vi "adapt_image_report.vi"() -> (3 "adapted image":T1)   [LabVIEW 2011]
doc: "Crops an image (original or captured) to cubic format (x-resolution = y-resolution) and applies a circular mask. Cropping and masking can be corrected using the crop-correction and mask-correction inputs.\n\nIf the input image is original (captured image set to FALSE) the image size will be adapted to match the size of the captured image and the image is flipped along the horizontal axis to account for the mirror image."
uses:
  <vilib>/vision/Image Controls.llb/IMAQ Image.ctl
  global_vars.vi
  <vilib>/vision/NI_Vision_Development_Module.lvlib
panel:
  out "cropped":T1(plugin-control)
  out "resized":T1(plugin-control)
  out "orig":T1(plugin-control)
  in  "File Path":path
  out "mirrored":T1(plugin-control)
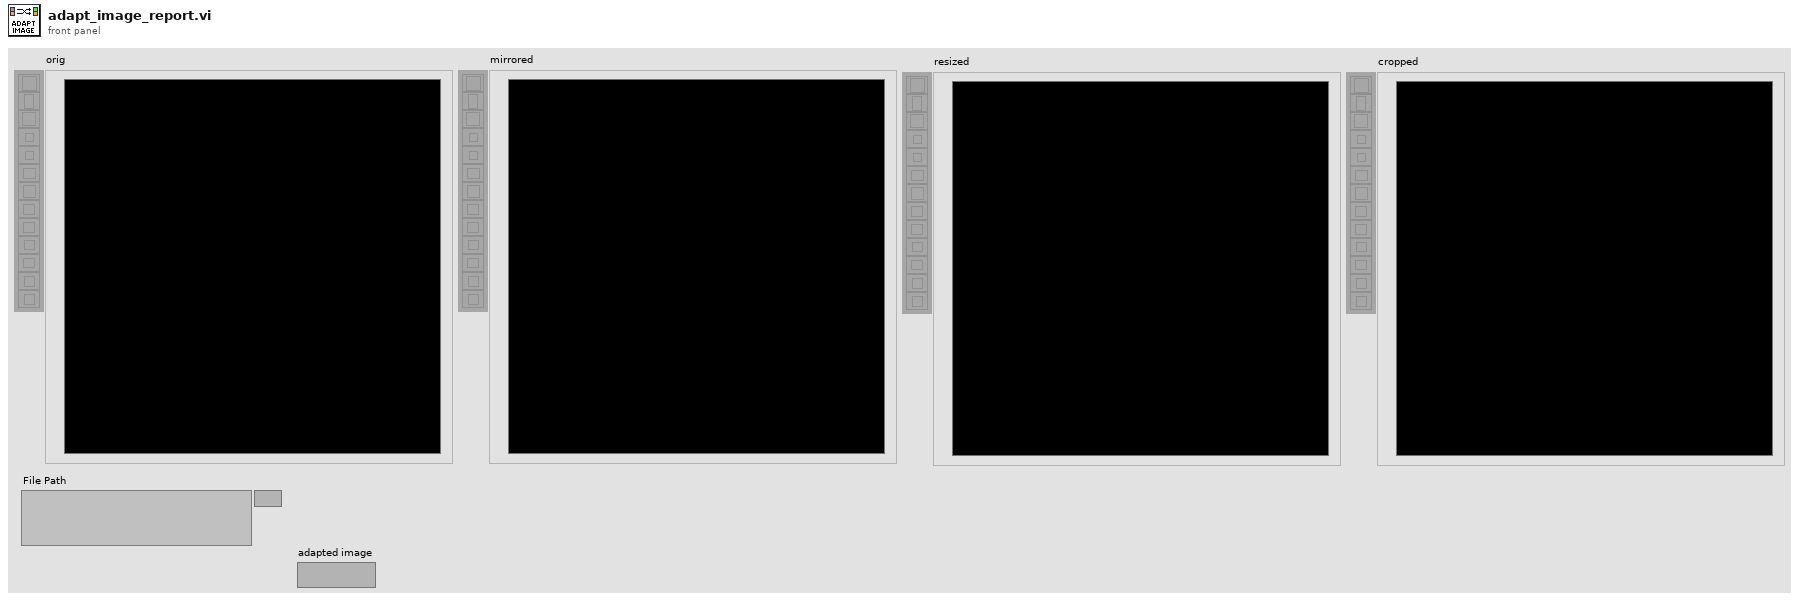
[diagram p1: front panel]
types:
  T1 = typedef "IMAQ Image.ctl" = refnum<image>
  T2 = typedef "Image Type" = u32
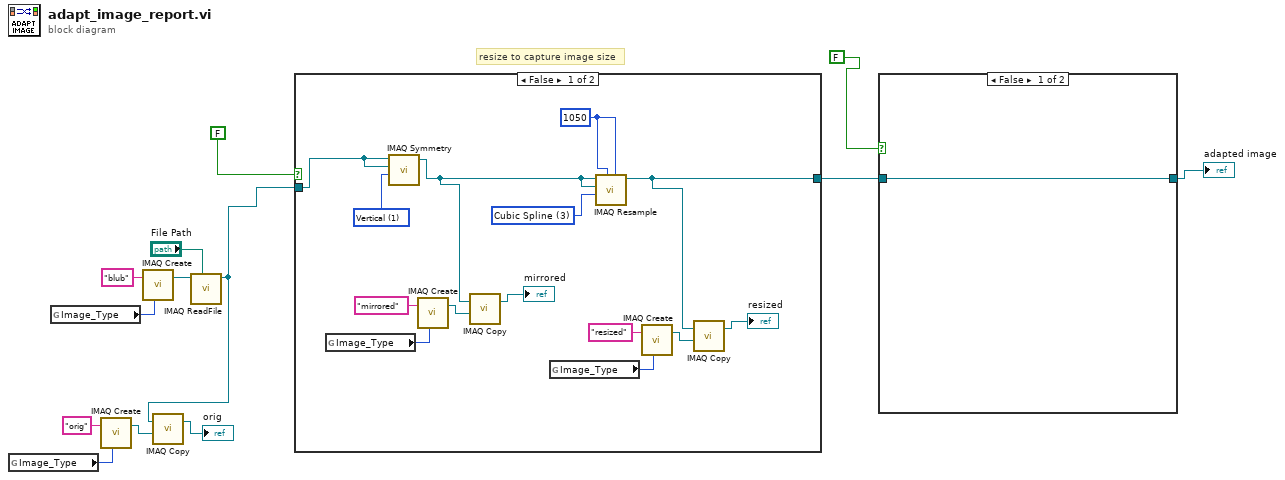
[diagram p0: block diagram]
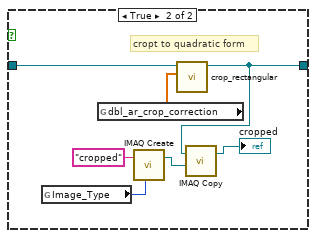
[diagram p2: hidden frame]
diagram:
  # "resize to capture image size"
  n1 = global read "global_vars.vi" "Image_Type"() -> (w2:T2)
  n2 = global read "global_vars.vi" "Image_Type"() -> (w9:T2)
  n3 = call "IMAQ Create"("Image Name"="orig", "Image Type"=w2) -> ("New Image"=w4:T1)  [unwired: 2 in, 2 out]
  n4 = call "IMAQ Create"("Image Name"="blub", "Image Type"=w9) -> ("New Image"=w7:T1)  [unwired: 2 in, 2 out]
  n5 = call "IMAQ ReadFile"("File Path"="File Path", "Image"=w7) -> ("Image Out"=w1:T1)  [unwired: 5 in, 4 out]
  n6 = call "IMAQ Copy"("Image Dst"=w4, "Image Src"=w1) -> ("Image Dst Out"=→"orig":T1)  [unwired: 4 in, 1 out]
  n7 = case shown="False" FALSE ("captured image?") {
    tunnel: [w15 w28] -> w13
    tunnel: w1 -> [w22 w28]
    frame False {
      w14 = 1050 ("captImage_X_Resolution")
      w26 = u32 1 items=["Horizontal", "Vertical", "Central", "1st Diagonal", "2nd Diagonal"] ("Type of Symmetry")
      w27 = u32 3 items=["Zero Order", "Bi-Linear", "Quadratic", "Cubic Spline"] ("Interpolation Type")
      n8 = global read "global_vars.vi" "Image_Type"() -> (w25:T2)
      n9 = call "IMAQ Symmetry"("Type of Symmetry"=w26, "Image Dst"=w22, "Image Src"=w22) -> ("Image Dst Out"=w20:T1)  [unwired: 2 in, 1 out]
      n10 = call "IMAQ Create"("Image Name"="mirrored", "Image Type"=w25) -> ("New Image"=w23:T1)  [unwired: 2 in, 2 out]
      n11 = call "IMAQ Copy"("Image Dst"=w23, "Image Src"=w20) -> ("Image Dst Out"=→"mirrored":T1)  [unwired: 4 in, 1 out]
      n12 = global read "global_vars.vi" "Image_Type"() -> (w16:T2)
      n13 = call "IMAQ Resample"("X Resolution"=w14, "Y Resolution"=w14, "Interpolation Type"=w27, "Image Dst"=w20, "Image Src"=w20) -> ("Image Dst Out"=w15:T1)  [unwired: 5 in, 1 out]
      n14 = call "IMAQ Create"("Image Name"="resized", "Image Type"=w16) -> ("New Image"=w18:T1)  [unwired: 2 in, 2 out]
      n15 = call "IMAQ Copy"("Image Dst"=w18, "Image Src"=w15) -> ("Image Dst Out"=→"resized":T1)  [unwired: 4 in, 1 out]
    }
    frame True {
    }
  }
  n16 = case shown="False" FALSE ("crop (TRUE)") {
    tunnel: w13 -> [w29 w36]
    tunnel: [w29 w30] -> w12
    frame False {
    }
    frame True {
      # "cropt to quadratic form"
      n17 = global read "global_vars.vi" "Image_Type"() -> (w31:T2)
      n18 = global read "global_vars.vi" "dbl_ar_crop_correction"() -> (w35:dbl[])
      n19 = call "IMAQ Create"("Image Name"="cropped", "Image Type"=w31) -> ("New Image"=w33:T1)  [unwired: 2 in, 2 out]
      n20 = call "crop_rectangular.vi"("dbl_ar_crop_correction"=w35, "image_in"=w36) -> ("cropped image out"=w30:T1)  [unwired: 8 in, 1 out]
      n21 = call "IMAQ Copy"("Image Dst"=w33, "Image Src"=w30) -> ("Image Dst Out"=→"cropped":T1)  [unwired: 4 in, 1 out]
    }
  }
  "adapted image" <- w12
